vi "Spline Torque Generator.vi"(11 "Spline Torque Parameters":T1) -> (3 "Desired Torque (Nm)":dbl[](array[numeric]))   [LabVIEW 2018, in "COBRA Torque Setpoint Generators Library.lvlib"]
uses:
  COBRA Torque Setpoint Generators Library.lvlib
  Target Spline Torque Parameters.ctl
  <vilib>/imath/engines/lvmath2/RunTimeEngine/Managers/WorkSpace/UID Generator.vi
  <vilib>/imath/engines/lvmath2/RunTimeEngine/BuiltInFunctions/length/NIMS_length(GV).vi
  <instcachedir>/0/NIMS_length(GV)_08A3D13377FD4E4B96F5795FBF3698FA.lvgen/NIMS_length(GV)_08A3D13377FD4E4B96F5795FBF3698FA_000.vi
  <vilib>/imath/engines/lvmath2/RunTimeEngine/BuiltInFunctions/zeros/NIMS_V=zeros(I32,I32).vi
  <vilib>/imathl/engines/lvmath/Functions/Error Handling/Create Error.vi
  <vilib>/imath/engines/lvmath2/RunTimeEngine/RangeToken/NIMS_Range_R2 - Integer.vi
  <instcachedir>/0/NIMS_Range_R2 - Integer_E35B921DECF84AADB7325A02D418BFCC.lvgen/NIMS_Range_R2 - Integer_E35B921DECF84AADB7325A02D418BFCC_000.vi
  <vilib>/imath/engines/lvmath2/RunTimeEngine/CommandStatement/MC_CommandStatement_break.vi
  <vilib>/imath/engines/lvmath2/RunTimeEngine/IndexRead/NIMS V(S).vi
  <instcachedir>/0/NIMS V(S)_0488751826AF41519A22953C041130DC.lvgen/NIMS V(S)_0488751826AF41519A22953C041130DC_000.vi
  <vilib>/imath/engines/lvmath2/RunTimeEngine/IndexReplace/NIMS V(S)=S.vi
  <instcachedir>/0/NIMS V(S)=S_420DA4522869420292A92FA3CC108C4E.lvgen/NIMS V(S)=S_420DA4522869420292A92FA3CC108C4E_000.vi
  <vilib>/imath/engines/lvmath2/RunTimeEngine/ErrorHandling/NIMS_Create Error From Enums.vi
  <vilib>/imath/engines/lvmath2/RunTimeEngine/IndexRead/NIMS V(R2).vi
  <instcachedir>/0/NIMS V(R2)_C76619605A0E4E9F8B2FA9389712AC47.lvgen/NIMS V(R2)_C76619605A0E4E9F8B2FA9389712AC47_000.vi
  <vilib>/imath/engines/lvmath2/RunTimeEngine/ArithmeticOperatorToken/NIMS_ArithmeticOperator_plus.vi
  <instcachedir>/0/NIMS_ArithmeticOperator_plus_DE670E32103C4C10ADF2A97367172B30.lvgen/NIMS_ArithmeticOperator_plus_DE670E32103C4C10ADF2A97367172B30_004.vi
  <vilib>/imath/engines/lvmath2/RunTimeEngine/ArithmeticOperatorToken/NIMS_ArithmeticOperator_times.vi
  <instcachedir>/0/NIMS_ArithmeticOperator_times_D7E4A7A4AD2C4409A0CE309D2741A5B4.lvgen/NIMS_ArithmeticOperator_times_D7E4A7A4AD2C4409A0CE309D2741A5B4_000.vi
  <vilib>/imath/engines/lvmath2/RunTimeEngine/BuiltInFunctions/diag/NIMS_diag.vi
  <instcachedir>/0/NIMS_diag_A176D428AACC4FD18ED77B06CA0A1FE1.lvgen/NIMS_diag_A176D428AACC4FD18ED77B06CA0A1FE1_003.vi
  <vilib>/imath/engines/lvmath2/RunTimeEngine/RowToken/NIMS_RowToken_CV_M.vi
  <instcachedir>/0/NIMS_RowToken_CV_M_38E0D26FC2F349BEAF24B377A79E2C1D.lvgen/NIMS_RowToken_CV_M_38E0D26FC2F349BEAF24B377A79E2C1D_000.vi
  <vilib>/imath/engines/lvmath2/RunTimeEngine/MatrixToken/NIMS_MatrixToken_M_RV.vi
  <instcachedir>/0/NIMS_MatrixToken_M_RV_284887C5C0C2478F8A28E9DD1730F3FE.lvgen/NIMS_MatrixToken_M_RV_284887C5C0C2478F8A28E9DD1730F3FE_001.vi
  <vilib>/imath/engines/lvmath2/RunTimeEngine/RowToken/NIMS_RowToken_M_CV.vi
  <instcachedir>/0/NIMS_RowToken_M_CV_6685E5BF66CC404F98B9B7041D694918.lvgen/NIMS_RowToken_M_CV_6685E5BF66CC404F98B9B7041D694918_000.vi
  <vilib>/imath/engines/lvmath2/RunTimeEngine/MatrixToken/NIMS_MatrixToken_RV_M.vi
  <instcachedir>/0/NIMS_MatrixToken_RV_M_6B17BADAEA014C61A1A547DE576F438D.lvgen/NIMS_MatrixToken_RV_M_6B17BADAEA014C61A1A547DE576F438D_000.vi
  <instcachedir>/0/NIMS_ArithmeticOperator_plus_DE670E32103C4C10ADF2A97367172B30.lvgen/NIMS_ArithmeticOperator_plus_DE670E32103C4C10ADF2A97367172B30_003.vi
  <vilib>/imath/engines/lvmath2/RunTimeEngine/IndexRead/NIMS M(S,$).vi
  <instcachedir>/0/NIMS M(S,$)_F24F360562DE41D8BE234322A2E15C65.lvgen/NIMS M(S,$)_F24F360562DE41D8BE234322A2E15C65_000.vi
  <vilib>/imath/engines/lvmath2/RunTimeEngine/BuiltInFunctions/size/NIMS_I32Row=size(GRow).vi
  <instcachedir>/0/NIMS_I32Row=size(GRow)_E5C05C6B13124B29B774CC4F993D3C59.lvgen/NIMS_I32Row=size(GRow)_E5C05C6B13124B29B774CC4F993D3C59_000.vi
  <vilib>/imath/engines/lvmath2/RunTimeEngine/BuiltInFunctions/zeros/NIMS_M=zeros(I32V).vi
  <vilib>/imath/engines/lvmath2/RunTimeEngine/IndexReplace/NIMS M(S,$)=M.vi
  <instcachedir>/0/NIMS M(S,$)=M_F300835DA1B94492A3F7D93B33F2631D.lvgen/NIMS M(S,$)=M_F300835DA1B94492A3F7D93B33F2631D_000.vi
  <vilib>/imath/engines/lvmath2/RunTimeEngine/IndexReplace/NIMS M(S,S)=S.vi
  <instcachedir>/0/NIMS M(S,S)=S_5DAF17B45D8A4C8588C7CF468644990A.lvgen/NIMS M(S,S)=S_5DAF17B45D8A4C8588C7CF468644990A_000.vi
  <vilib>/imath/engines/lvmath2/RunTimeEngine/ArithmeticOperatorToken/NIMS_ArithmeticOperator_leftdivmx.vi
  <instcachedir>/0/NIMS_ArithmeticOperator_leftdivmx_11C6409F72FD493AAD514540122EFCA2.lvgen/NIMS_ArithmeticOperator_leftdivmx_11C6409F72FD493AAD514540122EFCA2_000.vi
  <vilib>/imath/engines/lvmath2/RunTimeEngine/RunTimeType/NIMS_RunTimeType_From StrictType (excl LVString).vi
  <instcachedir>/0/NIMS_RunTimeType_From StrictType (excl LVString)_E7E34A65C99947108168652BAD14964D.lvgen/NIMS_RunTimeType_From StrictType (excl LVString)_E7E34A65C99947108168652BAD14964D_000.vi
  <vilib>/imath/engines/lvmath2/RunTimeEngine/LocalVariableDefStatement/MC_LocalVariableDefStatement_Display.vi
  <vilib>/imath/engines/lvmath2/RunTimeEngine/IndexRead/NIMS M(S).vi
  <instcachedir>/0/NIMS M(S)_B826C018497E4940AE96BD27B540B6FB.lvgen/NIMS M(S)_B826C018497E4940AE96BD27B540B6FB_000.vi
  <vilib>/imath/engines/lvmath2/RunTimeEngine/Managers/SymbolTable/Clear UID.vi
  <vilib>/imath/engines/lvmath2/RunTimeEngine/NodeEndStatement/NIMS_NodeEndStatement_Output.vi
  <instcachedir>/0/NIMS_NodeEndStatement_Output_53EC0D466D134D7ABD903AC30B43404B.lvgen/NIMS_NodeEndStatement_Output_53EC0D466D134D7ABD903AC30B43404B_005.vi
  <vilib>/imath/engines/lvmath2/RunTimeEngine/ErrorHandling/NIMS_Finalize Error.vi
  <vilib>/imath/engines/lvmath2/RunTimeEngine/Managers/SymbolTable/NIMS_WorkSpace.lvlib
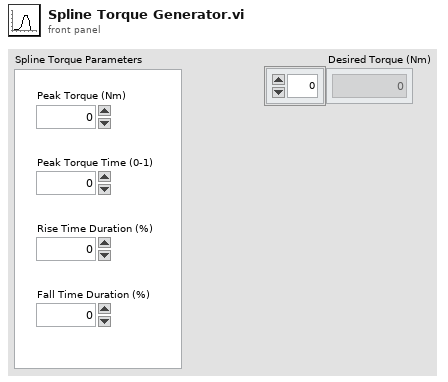
[diagram p1: front panel]
types:
  T1 = typedef "COBRA Torque Setpoint Generators Library.lvlib/Target Spline Torque Parameters.ctl" = cluster{"Peak Torque (Nm)":dbl, "Peak Torque Time (0-1)":dbl, "Rise Time Duration (%)":dbl, "Fall Time Duration (%)":dbl}
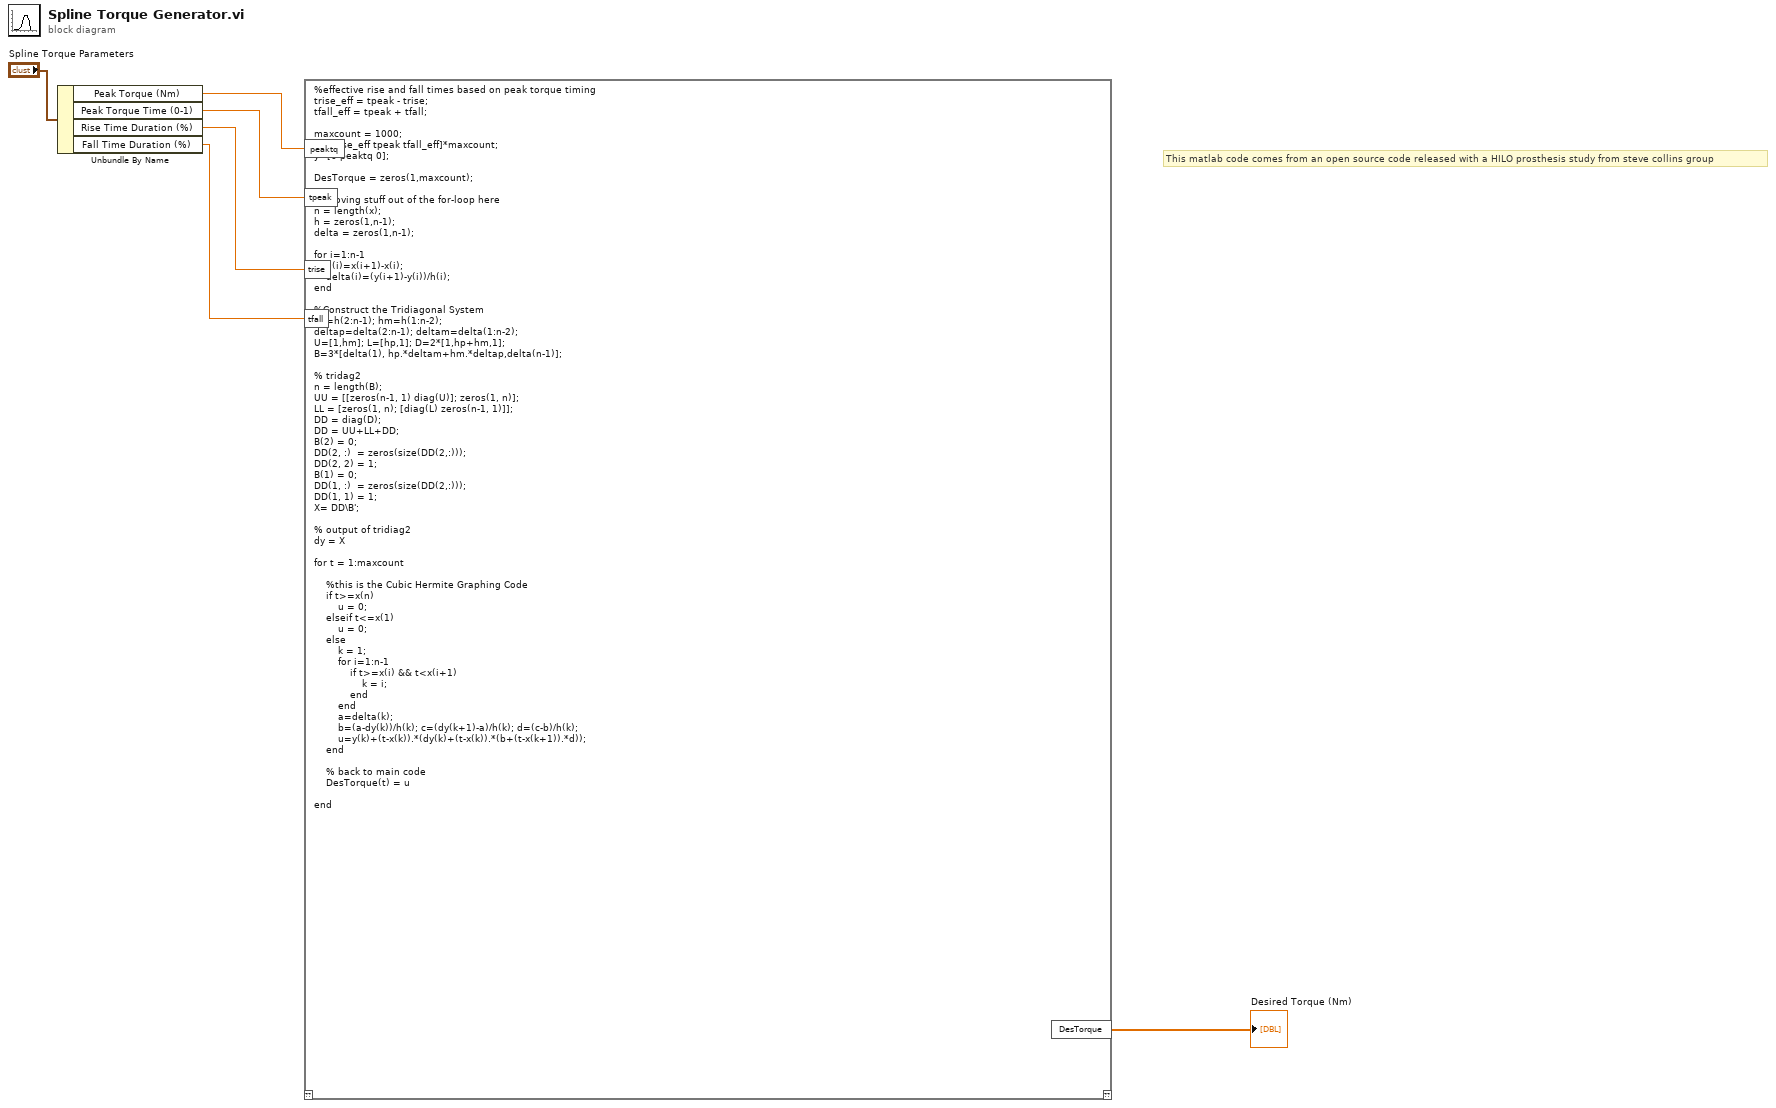
[diagram p0: block diagram]
diagram:
  # "This matlab code comes from an open source code released with a HILO prosthesis study from steve collins group"
  n1 = Unbundle By Name("Spline Torque Parameters") -> ("Peak Torque (Nm)"=w4:dbl, "Peak Torque Time (0-1)"=w3:dbl, "Rise Time Duration (%)"=w2:dbl, "Fall Time Duration (%)"=w1:dbl)
  n2 = mathscript code="%effective rise and fall times based on peak torque timing\ntrise_eff = tpeak - trise;\ntfall_eff = tpeak + tfall;\n\nmaxcount = 1000;\nx=[trise_eff tpeak tfall_eff]*maxcount;\ny=[0 peaktq 0];\n\nDesTorque = zeros(1,maxcount);\n\n% moving stuff out of the for-loop here\nn = length(x);\nh = zeros(1,n-1);\ndelta = zeros(1,n-1);\n\nfor i=1:n-1\n    h(i)=x(i+1)-x(i);\n    delta(i)=(y(i+1)-y(i))/h(i);\nend\n\n%Construct the Tridiagonal System\nhp=h(2:n-1); hm=h(1:n-2);\ndeltap=delta(2:n-1); deltam=delta(1:n-2);\nU=[1,hm]; L=[hp,1]; D=2*[1,hp+hm,1];\nB=3*[delta(1), hp.*deltam+hm.*deltap,delta(n-1)];\n\n% tridag2\nn = length(B);\nUU = [[zeros(n-1, 1) diag(U)]; zeros(1, n)];\nLL = [zeros(1, n); [diag(L) zeros(n-1, 1)]];\nDD = diag(D);\nDD = UU+LL+DD;\nB(2) = 0;\nDD(2, :)  = zeros(size(DD(2,:)));\nDD(2, 2) = 1;\nB(1) = 0;\nDD(1, :)  = zeros(size(DD(2,:)));\nDD(1, 1) = 1;\nX= DD\\B';\n    \n% output of tridiag2\ndy = X\n\nfor t = 1:maxcount\n\n    %this is the Cubic Hermite Graphing Code\n    if t>=x(n)\n        u = 0;\n    elseif t<=x(1)\n        u = 0;\n    else\n        k = 1;\n        for i=1:n-1\n            if t>=x(i) && t<x(i+1)\n                k = i;\n            end\n        end\n        a=delta(k);\n        b=(a-dy(k))/h(k); c=(dy(k+1)-a)/h(k); d=(c-b)/h(k);\n        u=y(k)+(t-x(k)).*(dy(k)+(t-x(k)).*(b+(t-x(k+1)).*d));\n    end\n\n    % back to main code\n    DesTorque(t) = u\n\nend"("peaktq"=w4, "tpeak"=w3, "trise"=w2, "tfall"=w1) -> ("DesTorque"=→"Desired Torque (Nm)":dbl[])  [unwired: 1 in, 1 out]
